vi "Voigt_Fit.vi"(5 "Freq_Data":dbl[](array[numeric]), 6 "Scptrm_Data":dbl[](array[numeric]), 7 "Freqs":T1={"Ffitlo / MHz"=70.0, "Fcentre / MHz"=80.0, "Ffithi / MHz"=90.0, "Lor HWHM / MHz"=2.6187499999999915, "Peak Est / nW"=0.0, "Gau stdev / MHz "=2.6187499999999915}) -> (0 "freq_fit_data":dbl[](array[numeric]), 1 "spctrm_fit_data":dbl[](array[numeric]), 2 "a_pars":dbl[](array[numeric])=[0.7072584069399376, 80.0, 1.7560129064005117], 3 "gof_stats":dbl[](array[numeric])=[3199.0, 1.0009386733416772, 0.954874518705434, 0.4817149539059473], 4 "Voigt LLM":dbl)   [LabVIEW 2020]
doc: "Fit a Voigt profile to measured LLM spectral data\n\nFreq_Data assumed in units of MHz\nSpctrm_Data assumed in units of dBm\nFfitlo, Ffithi in units of MHz must be inside range of Freq_Data\nFit_Data output in units of dBm\na_pars = [Amplitude, Centre Frequency [MHz], Lorentz HWHM [MHz], Gauss HWHM [MHz] ]\ngof_stats = [chi^{2}, chi^{2} / nu, R^{2}, gof probability]\nHWHM = Estimated LL [MHz]\n\nR. Sheehan 1 - 12 - 2021"
uses:
  Non_Lin_Fit/Release/Non_Lin_Fit.dll
panel:
  # "Amp. Par\n\nAOM Freq / MHz\n\nLorentzian HWHM / MHz\n\nGaussian Std. Dev.  / MHz"
  # "chi^{2} for the fit\n\nchi^{2} / nu\n\nR^{2}\n\nGOF"
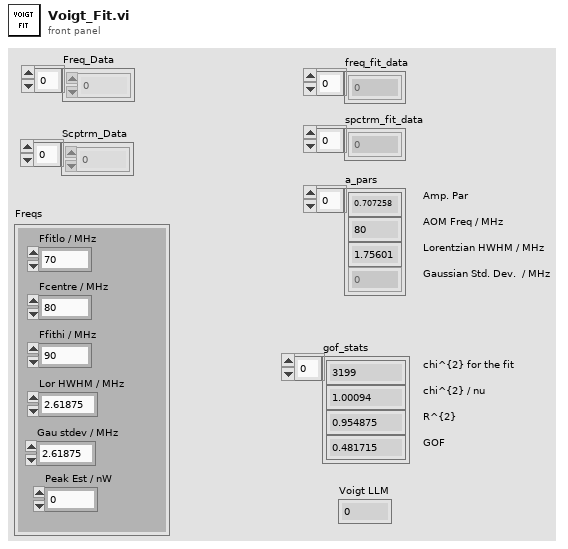
[diagram p1: front panel]
types:
  T1 = cluster{"Ffitlo / MHz":dbl, "Fcentre / MHz":dbl, "Ffithi / MHz":dbl, "Lor HWHM / MHz":dbl, "Peak Est / nW":dbl, "Gau stdev / MHz ":dbl}
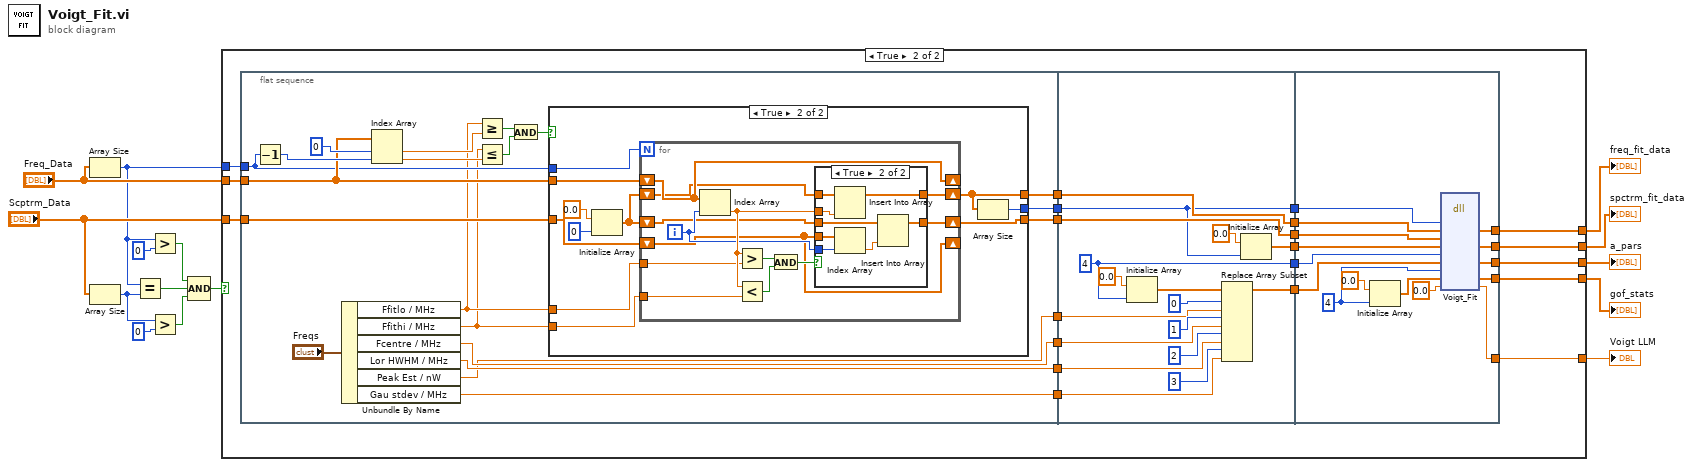
[diagram p0: block diagram]
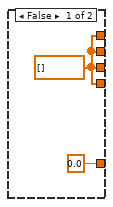
[diagram p2: hidden frame]
diagram:
  n1 = Array Size(array="Freq_Data") -> (size(s)=w10:i32)
  n2 = Array Size(array="Scptrm_Data") -> (size(s)=w11:i32)
  n3 = Equal?(x=w10, y=w11) -> (x = y?=w8:bool)
  n4 = Greater?(x=w10, y=0) -> (0:w9:bool)
  n5 = Greater?(x=w11, y=0) -> (0:w7:bool)
  n6 = Compound Arithmetic op=AND(w9, w8, w7) -> (w6:bool)
  n7 = case shown="True" w6 {
    tunnel: "Freq_Data" -> [_ w38]
    tunnel: "Scptrm_Data" -> [_ w37]
    tunnel: w10 -> [_ w36]
    tunnel: [w17 w24] -> w5
    tunnel: [w17 w23] -> w4
    tunnel: [w17 w22] -> w3
    tunnel: [w17 w21] -> w2
    tunnel: [0.0 ("HWHM") w19] -> w1
    frame False {
      w17 = dbl[] [] ("freq_data")
    }
    frame True {
      n8 = flat-sequence {
        tunnel: w38 -> [w51]
        tunnel: w37 -> [w50]
        tunnel: w36 -> [w49]
        tunnel: [w48] -> w35
        tunnel: [w47] -> w33
        tunnel: [w46] -> w31
        tunnel: [w42] -> w26
        tunnel: [w41] -> w25
        tunnel: [w40] -> w20
        tunnel: [w39] -> w18
        tunnel: w35 -> [w101]
        tunnel: [w106] -> w34
        tunnel: w33 -> [w106]
        tunnel: [w105] -> w32
        tunnel: w31 -> [w105]
        tunnel: [w104] -> w30
        tunnel: [w103] -> w29
        tunnel: [w102] -> w28
        tunnel: [w101] -> w27
        tunnel: w26 -> [w100]
        tunnel: w25 -> [w99]
        tunnel: w20 -> [w98]
        tunnel: w18 -> [w96]
        tunnel: w34 -> [w124]
        tunnel: w32 -> [w123]
        tunnel: w30 -> [w122]
        tunnel: w29 -> [w121]
        tunnel: w28 -> [w120]
        tunnel: w27 -> [w119]
        tunnel: [w118] -> w24
        tunnel: [w117] -> w23
        tunnel: [w116] -> w22
        tunnel: [w115] -> w21
        tunnel: [w114] -> w19
        frame #0 {
          n9 = Decrement(x=w49) -> (x-1=w56:i32)
          n10 = Unbundle By Name("Freqs") -> ("Ffitlo / MHz"=w44:dbl, "Ffithi / MHz"=w43:dbl, "Fcentre / MHz"=w42:dbl, "Lor HWHM / MHz"=w41:dbl, "Peak Est / nW"=w40:dbl, "Gau stdev / MHz"=w39:dbl)
          n11 = Index Array(array=w51, index #1=0 ("index"), index #2=w56) -> (element #1=w57:dbl, element #2=w55:dbl)
          n12 = Greater Or Equal?(x=w44, y=w57) -> (x >= y?=w54:bool)
          n13 = Less Or Equal?(x=w43, y=w55) -> (x <= y?=w53:bool)
          n14 = And(x=w54, y=w53) -> (x .and. y?=w52:bool)
          n15 = case shown="True" w52 {
            tunnel: w50 -> [w59 w72]
            tunnel: [w60 w68] -> w47
            tunnel: [w59 w67] -> w46
            tunnel: [w61 w66] -> w48
            tunnel: w44 -> [_ w65]
            tunnel: w51 -> [w60 w64]
            tunnel: w43 -> [_ w63]
            tunnel: w49 -> [w61 w62]
            frame False {
            }
            frame True {
              n16 = Initialize Array(0.0 ("element"), 0 ("dimension size")) -> (w69:dbl[])
              n17 = for {
                N: w62 -> [_]
                shift-right: [w85] -> _
                shift-left: w64 -> [w85]
                shift-right: [w79] -> _
                shift-left: w72 -> [w79]
                shift-right: [w77] -> w68
                shift-left: w69 -> [w78]
                shift-right: [w75] -> w67
                shift-left: w69 -> [w76]
                tunnel: w65 -> [w74]
                tunnel: w63 -> [w73]
                i -> [w80]
                n18 = Index Array(array=w85, index=w80) -> (element=w81:dbl)
                n19 = Greater?(x=w81, y=w74) -> (0:w84:bool)
                n20 = Less?(x=w81, y=w73) -> (x < y?=w83:bool)
                n21 = And(x=w84, y=w83) -> (x .and. y?=w82:bool)
                n22 = case shown="True" w82 {
                  tunnel: w81 -> [_ w91]
                  tunnel: w80 -> [_ w95]
                  tunnel: w79 -> [_ w94]
                  tunnel: w78 -> [w87 w93]
                  tunnel: [w87 w92] -> w77
                  tunnel: w76 -> [w86 w90]
                  tunnel: [w86 w89] -> w75
                  frame False {
                  }
                  frame True {
                    n23 = Insert Into Array(array=w93, new element=w91) -> (w92:dbl[])  [unwired: 1 in]
                    n24 = Index Array(array=w94, index=w95) -> (element=w88:dbl)
                    n25 = Insert Into Array(array=w90, new element=w88) -> (w89:dbl[])  [unwired: 1 in]
                  }
                }
              }
              n26 = Array Size(array=w68) -> (size(s)=w66:i32)
            }
          }
        }
        frame #1 {
          w102 = 4 ("Npars")
          n27 = Initialize Array(0.0 ("element"), w102) -> (w112:dbl[])
          n28 = Replace Array Subset(array=w112, new element #1=w98, index #1=0 ("index"), new element #2=w100, index #2=1 ("index"), new element #3=w99, index #3=2 ("index"), new element #4=w96, index #4=3 ("index")) -> (w103:dbl[])
          n29 = Initialize Array(0.0 ("element"), w101) -> (w104:dbl[])
        }
        frame #2 {
          w127 = 4 ("Nstats")
          n30 = Initialize Array(0.0 ("element"), w127) -> (w126:dbl[])
          n31 = dll-call lib="C:/Users/robertsheehan/Programming/C++/Fitting/Non_Lin_Fit/Release/Non_Lin_Fit.dll" fn="Voigt_Fit"("n_data"=w119, "freq_data"=w124, "spctrm_data"=w123, "fit_data"=w122, "n_pars"=w120, "a_pars"=w121, "n_stats"=w127, "gof_stats"=w126, "HWHM"=0.0) -> ("freq_data"=w118:dbl[], "fit_data"=w117:dbl[], "a_pars"=w116:dbl[], "gof_stats"=w115:dbl[], "HWHM"=w114:dbl)  [unwired: 8 in, 2 out]
        }
      }
    }
  }
  "freq_fit_data" <- w5
  "spctrm_fit_data" <- w4
  "a_pars" <- w3
  "gof_stats" <- w2
  "Voigt LLM" <- w1
